vi "TEST - Initialize Array to Variant Array.vi"(8 "error in (no error)":errorcluster) -> (0 "error out":errorcluster, 2 "Pass?":bool=TRUE)   [LabVIEW 2009]
doc: "This VI template can be used for the functional testing of VIs; this implementation includes handling for the testing of polymorphic VIs, and the polymorphic elements should be removed if not needed.\n\nCoded by Douglas A. Femec, January 24, 2006.\n\nCopyright (c) 2005-2006 MKS Instruments, Inc.\nAll rights reserved."
uses:
  TEST - Initialize Array from Array - Inputs.ctl
  Polymorphizer+ Data Type.ctl
  TEST - Initialize Array from Array - Outputs.ctl
  source/library/Initialize Array from Array/Initialize 1D Array (Variant) from 1D Array (EXT).vi
  source/library/Initialize Array from Array/Initialize 2D Array (Variant) from 2D Array (EXT).vi
  source/library/Initialize Array from Array/Initialize 1D Array (Variant) from 1D Array (I64).vi
  source/library/Initialize Array from Array/Initialize 2D Array (Variant) from 2D Array (I64).vi
  source/library/Initialize Array from Array/Initialize 1D Array (Variant) from 1D Array (U64).vi
  source/library/Initialize Array from Array/Initialize 1D Array (Variant) from 1D Array (DBL).vi
  source/library/Initialize Array from Array/Initialize 2D Array (Variant) from 2D Array (DBL).vi
  source/library/Initialize Array from Array/Initialize 1D Array (Variant) from 1D Array (SGL).vi
  source/library/Initialize Array from Array/Initialize 2D Array (Variant) from 2D Array (SGL).vi
  source/library/Initialize Array from Array/Initialize 1D Array (Variant) from 1D Array (I32).vi
  source/library/Initialize Array from Array/Initialize 2D Array (Variant) from 2D Array (I32).vi
  source/library/Initialize Array from Array/Initialize 1D Array (Variant) from 1D Array (I16).vi
  source/library/Initialize Array from Array/Initialize 2D Array (Variant) from 2D Array (I16).vi
  source/library/Initialize Array from Array/Initialize 1D Array (Variant) from 1D Array (I8).vi
  source/library/Initialize Array from Array/Initialize 2D Array (Variant) from 2D Array (I8).vi
  source/library/Initialize Array from Array/Initialize 1D Array (Variant) from 1D Array (U32).vi
  source/library/Initialize Array from Array/Initialize 2D Array (Variant) from 2D Array (U32).vi
  source/library/Initialize Array from Array/Initialize 1D Array (Variant) from 1D Array (U16).vi
  source/library/Initialize Array from Array/Initialize 2D Array (Variant) from 2D Array (U16).vi
  source/library/Initialize Array from Array/Initialize 1D Array (Variant) from 1D Array (U8).vi
  source/library/Initialize Array from Array/Initialize 2D Array (Variant) from 2D Array (U8).vi
  source/library/Initialize Array from Array/Initialize 1D Array (Variant) from 1D Array (Boolean).vi
  source/library/Initialize Array from Array/Initialize 2D Array (Variant) from 2D Array (Boolean).vi
  source/library/Initialize Array from Array/Initialize 1D Array (Variant) from 1D Array (String).vi
  source/library/Initialize Array from Array/Initialize 2D Array (Variant) from 2D Array (String).vi
  source/library/Initialize Array from Array/Initialize 1D Array (Variant) from 1D Array (Path).vi
  source/library/Initialize Array from Array/Initialize 2D Array (Variant) from 2D Array (Path).vi
  source/library/Initialize Array from Array/Initialize 1D Array (Variant) from 1D Array (Variant).vi
  source/library/Initialize Array from Array/Initialize 2D Array (Variant) from 2D Array (Variant).vi
panel:
  out "Generated Outputs":T1[][](array[typedef]) {"1D Array" format="%.2f"; "2D Array" format="%.2f"}
  in  "Expected Outputs":T1[](array[typedef])=[{"Description"="Expect empty arrays", "1D Array"=[], "2D Array"=[]}, {"Description"="Expect 1-element arrays", "1D Array"=[1.0], "2D Array"=[[1.0]]}, {"Description"="Expect 1-row arrays", "1D Array"=[1.0], "2D Array"=[[1.0, 1.0]]}, {"Description"="Expect 1-column arrays", "1D Array"=[1.0], "2D Array"=[[1.0], [1.0], [1.0], [1.0]]}, {"Description"="Expect 2-columns, 4-rows arrays", "1D Array"=[1.0, 1.0, 1.0, 1.0], "2D Array"=[[1.0, 1.0], [1.0, 1.0], [1.0, 1.0], [1.0, 1.0]]}] {"1D Array" format="%.2f"; "2D Array" format="%.2f"}
  in  "Inputs":T2[](array[typedef])=[{"Description"="Empty arrays", "Data Types to Test"=[enum."EXT", enum."DBL", enum."SGL", enum."I32", enum."I16", enum."I8", enum."U32", enum."U16", enum."U8", enum."Boolean", enum."String", enum."Path", enum."Variant", enum."I64", enum."U64"], "1D Array"=[], "2D Array"=[]}, {"Description"="1-Element arrays", "Data Types to Test"=[enum."EXT", enum."DBL", enum."SGL", enum."I32", enum."I16", enum."I8", enum."U32", enum."U16", enum."U8", enum."Boolean", enum."String", enum."Path", enum."Variant", enum."I64", enum."U64"], "1D Array"=[1.0], "2D Array"=[[1.0]]}, {"Description"="1-Row arrays", "Data Types to Test"=[enum."EXT", enum."DBL", enum."SGL", enum."I32", enum."I16", enum."I8", enum."U32", enum."U16", enum."U8", enum."Boolean", enum."String", enum."Path", enum."Variant", enum."I64", enum."U64"], "1D Array"=[1.0], "2D Array"=[[1.0, 1.0]]}, {"Description"="1-Column arrays", "Data Types to Test"=[enum."EXT", enum."DBL", enum."SGL", enum."I32", enum."I16", enum."I8", enum."U32", enum."U16", enum."U8", enum."Boolean", enum."String", enum."Path", enum."Variant", enum."I64", enum."U64"], "1D Array"=[1.0], "2D Array"=[[1.0], [1.0], [1.0], [1.0]]}, {"Description"="2-Columns, 4-rows arrays", "Data Types to Test"=[enum."EXT", enum."DBL", enum."SGL", enum."I32", enum."I16", enum."I8", enum."U32", enum."U16", enum."U8", enum."Boolean", enum."String", enum."Path", enum."Variant", enum."I64", enum."U64"], "1D Array"=[1.0, 1.0, 1.0, 1.0], "2D Array"=[[1.0, 1.0], [1.0, 1.0], [1.0, 1.0], [1.0, 1.0]]}] {"1D Array" format="%.2f"; "2D Array" format="%.2f"}
  # "Copyright (c) 2005-2006 MKS Instruments, Inc.\nAll rights reserved."
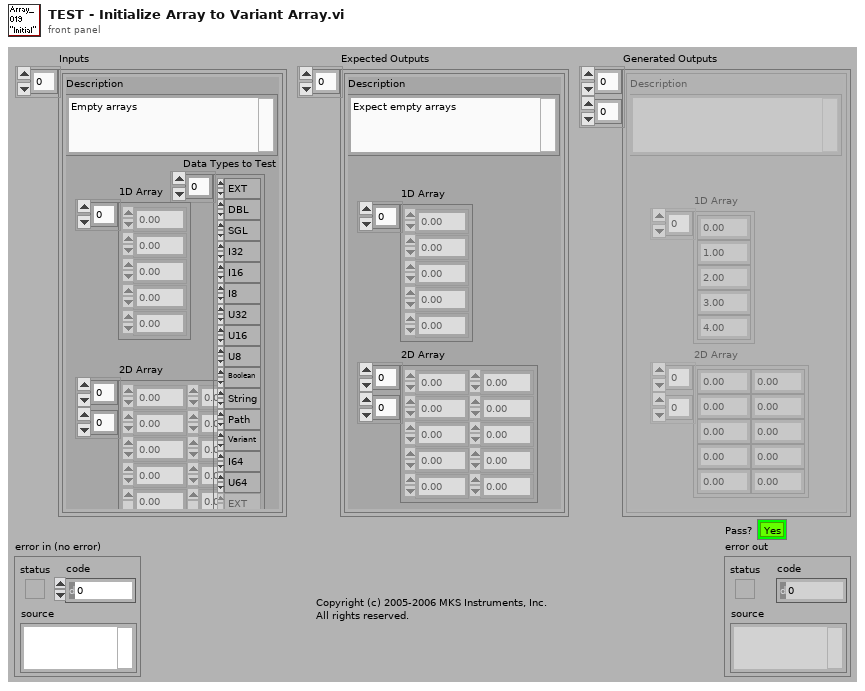
[diagram p1: front panel]
types:
  T1 = typedef "TEST - Initialize Array from Array - Outputs.ctl" = cluster{"Description":string, "1D Array":sgl[], "2D Array":sgl[][]}
  T2 = typedef "TEST - Initialize Array from Array - Inputs.ctl" = cluster{"Description":string, "Data Types to Test":T3[], "1D Array":sgl[], "2D Array":sgl[][]}
  T3 = typedef "Polymorphizer+ Data Type.ctl" = enum16{"EXT", "DBL", "SGL", "I32", "I16", "I8", "U32", "U16", "U8", "CXT", "CDB", "CSG", "Boolean", "String", "Path", "Variant", "CTL-REF", "GEN-REF", "GObj-REF", "VI-REF", "ENUM", "ERR", "FILE-REF", "MENU-REF", "MENU-RING", "PICT-RING", "TXT&PICT-RING", "TXT-RING", "I64", "U64", "LabVIEW Object"}
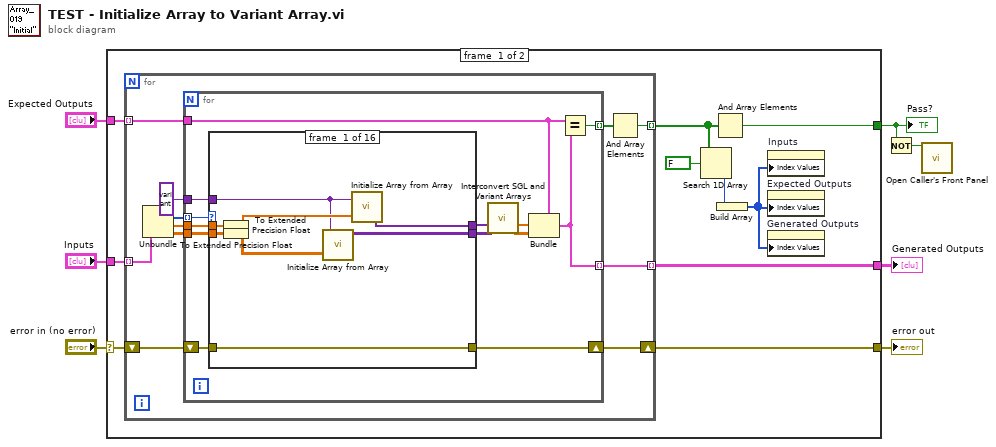
[diagram p0: block diagram]
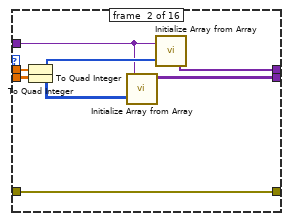
[diagram p2: hidden frame]
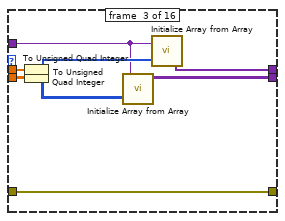
[diagram p3: hidden frame]
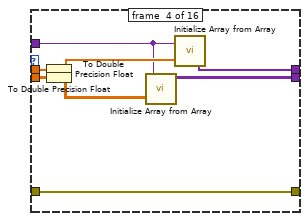
[diagram p4: hidden frame]
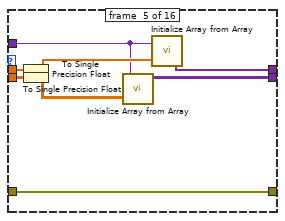
[diagram p5: hidden frame]
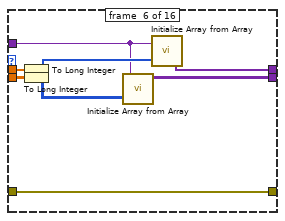
[diagram p6: hidden frame]
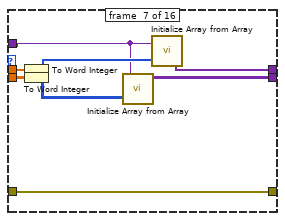
[diagram p7: hidden frame]
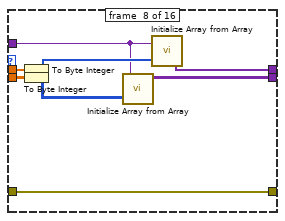
[diagram p8: hidden frame]
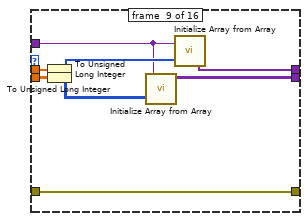
[diagram p9: hidden frame]
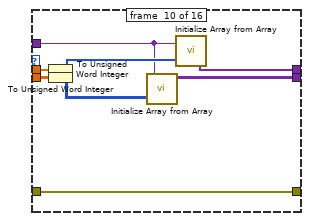
[diagram p10: hidden frame]
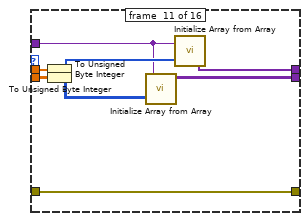
[diagram p11: hidden frame]
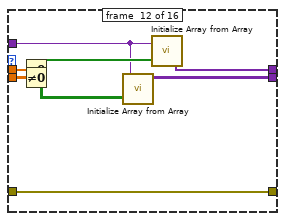
[diagram p12: hidden frame]
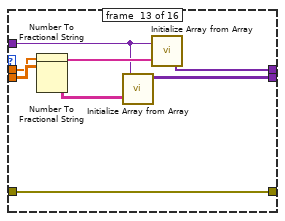
[diagram p13: hidden frame]
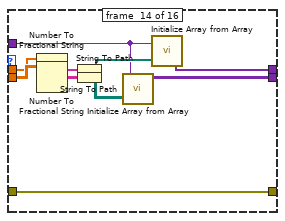
[diagram p14: hidden frame]
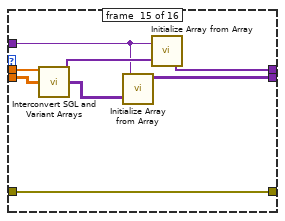
[diagram p15: hidden frame]
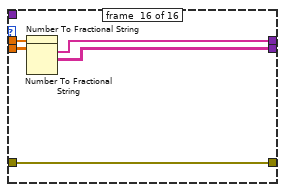
[diagram p16: hidden frame]
diagram:
  n1 = case shown="No Error" "error in (no error)" {
    selector: "error in (no error)" -> [w16 w169]
    tunnel: [w17 w169] -> w6
    tunnel: "Expected Outputs" -> [w14 _]
    tunnel: "Inputs" -> [w15 _]
    tunnel: [w13 _] -> w3
    tunnel: [w12 _] -> w1
    frame #0 {
      n2 = for {
        shift-right: [w23] -> w17
        shift-left: w16 -> [w24]
        tunnel: w15 -> [w25] mode=indexing
        tunnel: w14 -> [w28] mode=indexing
        tunnel: [w27] -> w13 mode=indexing
        tunnel: [w22] -> w11 mode=indexing
        n3 = Unbundle(w25) -> ("Data Types to Test"=w19:T3[], "1D Array"=w20:sgl[], "2D Array"=w21:sgl[][])  [unwired: 1 out]
        n4 = for {
          tunnel: w28 -> [w41]
          tunnel: [w39] -> w27 mode=indexing
          tunnel: [w40] -> w26 mode=indexing
          shift-right: [w36] -> w23
          shift-left: w24 -> [w37]
          tunnel: w19 -> [w38] mode=indexing
          tunnel: w20 -> [w34]
          tunnel: w21 -> [w33]
          tunnel: variant(i8 1) ("Variant") -> [w35]
          n5 = case shown="\"U64\"" w38 {
            tunnel: w34 -> [w48 w56 w64 w72 w80 w88 w96 w104 w112 w120 w128 w136 w144 w152 w161 w164]
            tunnel: [w46 w54 w62 w70 w75 w84 w91 w99 w107 w115 w126 w131 w139 w147 w157 w166] -> w32
            tunnel: [w45 w53 w61 w67 w78 w86 w94 w102 w110 w118 w125 w130 w138 w146 w156 w167] -> w31
            tunnel: w33 -> [w49 w57 w65 w73 w81 w89 w97 w105 w113 w121 w129 w137 w145 w154 w162 w165]
            tunnel: w37 -> [w47 w55 w63 w71 w79 w87 w95 w103 w111 w119 w127 w135 w143 w151 w163 w168]
            tunnel: [w47 w55 w63 w71 w79 w87 w95 w103 w111 w119 w127 w135 w143 w151 w163 w168] -> w36
            tunnel: w35 -> [w42 w50 w58 w66 w74 w82 w90 w98 w106 w114 w122 w132 w140 w148 w158 _]
            frame #0 {
              n6 = To Extended Precision Float(1:w48) -> (0:w43:ext[])
              n7 = To Extended Precision Float(1:w49) -> (0:w44:ext[][])
              n8 = call-poly "Initialize Array from Array.vi"("Input Array"=w44, "Element Data"=w42) -> ("Output Array"=w45:variant[][])
              n9 = call-poly "Initialize Array from Array.vi"("Input Array"=w43, "Element Data"=w42) -> ("Output Array"=w46:variant[])
            }
            frame #1 {
              n10 = To Quad Integer(1:w56) -> (0:w51:i64[])
              n11 = To Quad Integer(1:w57) -> (0:w52:i64[][])
              n12 = call-poly "Initialize Array from Array.vi"("Input Array"=w52, "Element Data"=w50) -> ("Output Array"=w53:variant[][])
              n13 = call-poly "Initialize Array from Array.vi"("Input Array"=w51, "Element Data"=w50) -> ("Output Array"=w54:variant[])
            }
            frame #2 {
              n14 = To Unsigned Quad Integer(1:w64) -> (0:w59:u64[])
              n15 = To Unsigned Quad Integer(1:w65) -> (0:w60:u64[][])
              n16 = call-poly "Initialize Array from Array.vi"("Input Array"=w60, "Element Data"=w58) -> ("Output Array"=w61:variant[][])
              n17 = call-poly "Initialize Array from Array.vi"("Input Array"=w59, "Element Data"=w58) -> ("Output Array"=w62:variant[])
            }
            frame #3 {
              n18 = To Double Precision Float(number=w72) -> (double precision float=w69:dbl[])
              n19 = To Double Precision Float(number=w73) -> (double precision float=w68:dbl[][])
              n20 = call-poly "Initialize Array from Array.vi"("Input Array"=w68, "Element Data"=w66) -> ("Output Array"=w67:variant[][])
              n21 = call-poly "Initialize Array from Array.vi"("Input Array"=w69, "Element Data"=w66) -> ("Output Array"=w70:variant[])
            }
            frame #4 {
              n22 = To Single Precision Float(number=w80) -> (single precision float=w77:sgl[])
              n23 = To Single Precision Float(number=w81) -> (single precision float=w76:sgl[][])
              n24 = call-poly "Initialize Array from Array.vi"("Input Array"=w76, "Element Data"=w74) -> ("Output Array"=w78:variant[][])
              n25 = call-poly "Initialize Array from Array.vi"("Input Array"=w77, "Element Data"=w74) -> ("Output Array"=w75:variant[])
            }
            frame #5 {
              n26 = To Long Integer(number=w88) -> (32bit integer=w83:i32[])
              n27 = To Long Integer(number=w89) -> (32bit integer=w85:i32[][])
              n28 = call-poly "Initialize Array from Array.vi"("Input Array"=w85, "Element Data"=w82) -> ("Output Array"=w86:variant[][])
              n29 = call-poly "Initialize Array from Array.vi"("Input Array"=w83, "Element Data"=w82) -> ("Output Array"=w84:variant[])
            }
            frame #6 {
              n30 = To Word Integer(number=w96) -> (16bit integer=w93:i16[])
              n31 = To Word Integer(number=w97) -> (16bit integer=w92:i16[][])
              n32 = call-poly "Initialize Array from Array.vi"("Input Array"=w92, "Element Data"=w90) -> ("Output Array"=w94:variant[][])
              n33 = call-poly "Initialize Array from Array.vi"("Input Array"=w93, "Element Data"=w90) -> ("Output Array"=w91:variant[])
            }
            frame #7 {
              n34 = To Byte Integer(number=w104) -> (8bit integer=w101:i8[])
              n35 = To Byte Integer(number=w105) -> (8bit integer=w100:i8[][])
              n36 = call-poly "Initialize Array from Array.vi"("Input Array"=w100, "Element Data"=w98) -> ("Output Array"=w102:variant[][])
              n37 = call-poly "Initialize Array from Array.vi"("Input Array"=w101, "Element Data"=w98) -> ("Output Array"=w99:variant[])
            }
            frame #8 {
              n38 = To Unsigned Long Integer(number=w112) -> (unsigned 32bit integer=w109:u32[])
              n39 = To Unsigned Long Integer(number=w113) -> (unsigned 32bit integer=w108:u32[][])
              n40 = call-poly "Initialize Array from Array.vi"("Input Array"=w108, "Element Data"=w106) -> ("Output Array"=w110:variant[][])
              n41 = call-poly "Initialize Array from Array.vi"("Input Array"=w109, "Element Data"=w106) -> ("Output Array"=w107:variant[])
            }
            frame #9 {
              n42 = To Unsigned Word Integer(number=w120) -> (unsigned 16bit integer=w117:u16[])
              n43 = To Unsigned Word Integer(number=w121) -> (unsigned 16bit integer=w116:u16[][])
              n44 = call-poly "Initialize Array from Array.vi"("Input Array"=w116, "Element Data"=w114) -> ("Output Array"=w118:variant[][])
              n45 = call-poly "Initialize Array from Array.vi"("Input Array"=w117, "Element Data"=w114) -> ("Output Array"=w115:variant[])
            }
            frame #10 {
              n46 = To Unsigned Byte Integer(number=w128) -> (unsigned 8bit integer=w123:u8[])
              n47 = To Unsigned Byte Integer(number=w129) -> (unsigned 8bit integer=w124:u8[][])
              n48 = call-poly "Initialize Array from Array.vi"("Input Array"=w124, "Element Data"=w122) -> ("Output Array"=w125:variant[][])
              n49 = call-poly "Initialize Array from Array.vi"("Input Array"=w123, "Element Data"=w122) -> ("Output Array"=w126:variant[])
            }
            frame #11 {
              n50 = Not Equal To 0?(x=w136) -> (x != 0?=w134:bool[])
              n51 = Not Equal To 0?(x=w137) -> (x != 0?=w133:bool[][])
              n52 = call-poly "Initialize Array from Array.vi"("Input Array"=w133, "Element Data"=w132) -> ("Output Array"=w130:variant[][])
              n53 = call-poly "Initialize Array from Array.vi"("Input Array"=w134, "Element Data"=w132) -> ("Output Array"=w131:variant[])
            }
            frame #12 {
              n54 = Number To Fractional String(number=w144) -> (F-format string=w142:string[])  [unwired: 3 in]
              n55 = Number To Fractional String(number=w145) -> (F-format string=w141:string[][])  [unwired: 3 in]
              n56 = call-poly "Initialize Array from Array.vi"("Input Array"=w141, "Element Data"=w140) -> ("Output Array"=w138:variant[][])
              n57 = call-poly "Initialize Array from Array.vi"("Input Array"=w142, "Element Data"=w140) -> ("Output Array"=w139:variant[])
            }
            frame #13 {
              n58 = Number To Fractional String(number=w152) -> (F-format string=w153:string[])  [unwired: 3 in]
              n59 = Number To Fractional String(number=w154) -> (F-format string=w155:string[][])  [unwired: 3 in]
              n60 = String To Path(string=w153) -> (path=w150:path[])
              n61 = String To Path(string=w155) -> (path=w149:path[][])
              n62 = call-poly "Initialize Array from Array.vi"("Input Array"=w149, "Element Data"=w148) -> ("Output Array"=w146:variant[][])
              n63 = call-poly "Initialize Array from Array.vi"("Input Array"=w150, "Element Data"=w148) -> ("Output Array"=w147:variant[])
            }
            frame #14 {
              n64 = call "Interconvert SGL and Variant Arrays.vi"("SGL 1D Array In"=w161, "SGL 2D Array In"=w162) -> ("Variant 1D Array Out"=w160:variant[], "Variant 2D Array Out"=w159:variant[][])  [unwired: 9 in, 3 out]
              n65 = call-poly "Initialize Array from Array.vi"("Input Array"=w159, "Element Data"=w158) -> ("Output Array"=w156:variant[][])
              n66 = call-poly "Initialize Array from Array.vi"("Input Array"=w160, "Element Data"=w158) -> ("Output Array"=w157:variant[])
            }
            frame #15 {
              n67 = Number To Fractional String(number=w164) -> (F-format string=w166:string[])  [unwired: 3 in]
              n68 = Number To Fractional String(number=w165) -> (F-format string=w167:string[][])  [unwired: 3 in]
            }
          }
          n69 = call "Interconvert SGL and Variant Arrays.vi"("Variant 1D Array In"=w32, "Variant 2D Array In"=w31) -> ("SGL 1D Array Out"=w30:sgl[], "SGL 2D Array Out"=w29:sgl[][])  [unwired: 9 in, 3 out]
          n70 = Bundle(cluster=w41, "1D Array"=w30, "2D Array"=w29) -> (w39:T1)  [unwired: 1 in]
          n71 = Equal?(x=w41, y=w39) -> (x = y?=w40:bool)
        }
        n72 = And Array Elements(Boolean array=w26) -> (logical AND=w22:bool)
      }
      n73 = Search 1D Array(1D array=w11, element=FALSE) -> (index of element=w9:i32)  [unwired: 1 in]
      n74 = And Array Elements(Boolean array=w11) -> (logical AND=w12:bool)
      n75 = Build Array(w9) -> (w8:i32[])
      n76 = property on="Inputs" class="Arr (strict)"("Index Values"=w8) -> ()  [unwired: 2 in, 2 out]
      n77 = property on="Expected Outputs" class="Arr (strict)"("Index Values"=w8) -> ()  [unwired: 2 in, 2 out]
      n78 = property on="Generated Outputs" class="Arr (strict)"("Index Values"=w8) -> ()  [unwired: 2 in, 2 out]
    }
    frame #1 {
    }
  }
  "error out" <- w6
  "Pass?" <- w1
  "Generated Outputs" <- w3
  n79 = Not(x=w1) -> (.not. x?=w2:bool)
  n80 = call "Open Caller's Front Panel.vi"("Open?"=w2) -> ()  [unwired: 14 in, 1 out]
